vi "带表头写入EXCEL并加入时间量.vi"() -> ()   [LabVIEW 2014]
panel:
  out "保存的路径":path
  out "序号":dbl format="%06.0f"
  in  "起始号":dbl format="%0#6.0p"
  in  "停止":bool
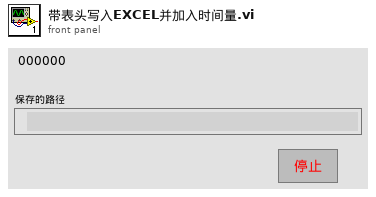
[diagram p1: front panel]
types:
  T1 = enum16{"open", "replace", "create", "open or create", "replace or create", "replace or create with confirmation"}
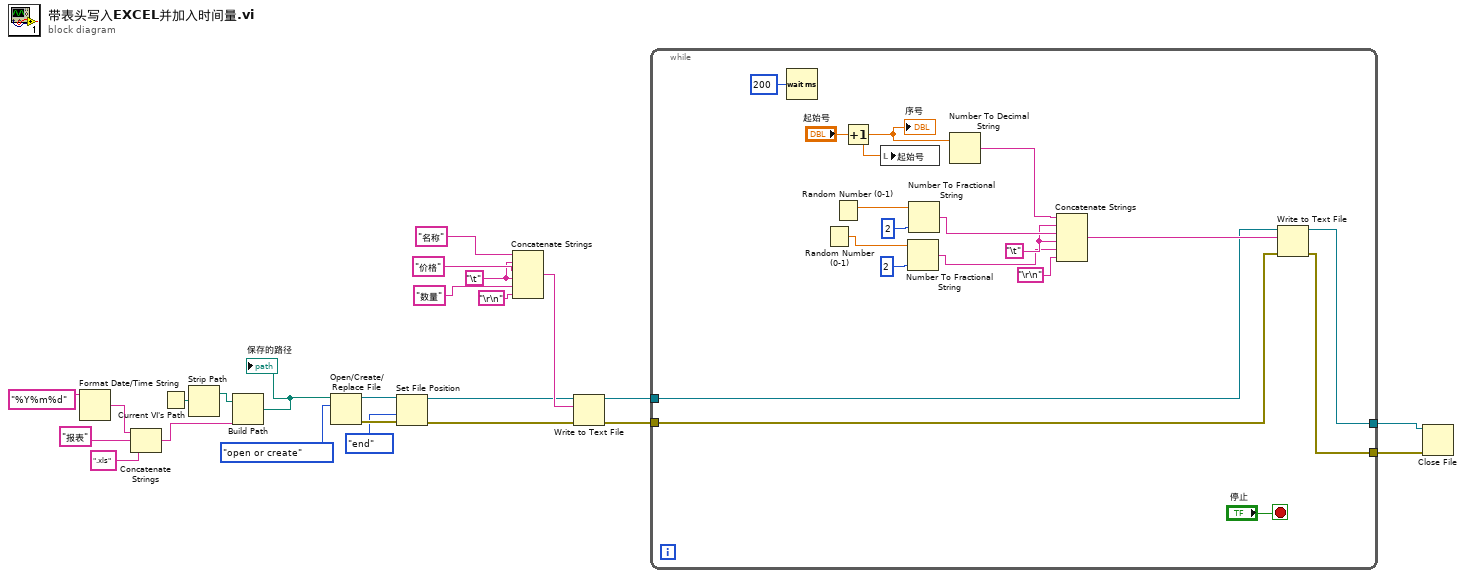
[diagram p0: block diagram]
diagram:
  w5 = "\t"
  n1 = Format Date/Time String(time format string (%c)="%Y%m%d" ("时间格式字符串(%c)")) -> (date/time string=w13:string)  [unwired: 2 in]
  n2 = Concatenate Strings(w13, "报表" ("名称或相对路径"), ".xls" ("字符串")) -> (w19:string)
  n3 = Current VI's Path() -> (path=w18:path)
  n4 = Strip Path(path=w18) -> (stripped path=w17:path)  [unwired: 1 out]
  n5 = Build Path(base path=w17, name or relative path=w19) -> (appended path=w12:path)
  "保存的路径" <- w12
  n6 = Open/Create/Replace File(file path (use dialog)=w12, operation (0:open)=T1."open or create" ("操作(0:open)")) -> (refnum out=w11:refnum<file>, error out=w21:errorcluster)  [unwired: 4 in, 1 out]
  n7 = Set File Position(refnum=w11, from (0:start)=enum16{"start", "end", "current"}."end" ("自（0:起始）"), error in=w21) -> (refnum out=w4:refnum<file>, error out=w3:errorcluster)  [unwired: 1 in]
  n8 = Concatenate Strings("名称" ("字符串"), w5, "价格" ("字符串"), w5, "数量" ("字符串"), "\r\n") -> (w6:string)
  n9 = Write to Text File(file (use dialog)=w4, text=w6, error in=w3) -> (refnum out=w2:refnum<file>, error out=w1:errorcluster)  [unwired: 1 in, 1 out]
  n10 = while {
    tunnel: [w28] -> w24
    tunnel: [w27] -> w23
    tunnel: w2 -> [w26]
    tunnel: w1 -> [w25]
    stop <- "停止" stop-if-true
    w31 = "\t"
    n11 = Wait (ms)(milliseconds to wait=u32 200 ("等待时间（毫秒）")) -> ()  [unwired: 1 out]
    n12 = Random Number (0-1)() -> (number: 0 to 1=w38:dbl)
    n13 = Random Number (0-1)() -> (number: 0 to 1=w36:dbl)
    n14 = Increment(x="起始号") -> (x+1=w34:dbl)
    "序号" <- w34
    n15 = local write "起始号"(w34) -> ()
    n16 = Number To Fractional String(number=w38, precision (6)=i16 2 ("精度(6)")) -> (F-format string=w30:string)  [unwired: 2 in]
    n17 = Number To Fractional String(number=w36, precision (6)=i16 2 ("精度(6)")) -> (F-format string=w32:string)  [unwired: 2 in]
    n18 = Number To Decimal String(number=w34) -> (decimal integer string=w33:string)  [unwired: 1 in]
    n19 = Concatenate Strings(w33, w31, w32, w31, w30, "\r\n") -> (w41:string)
    n20 = Write to Text File(file (use dialog)=w26, text=w41, error in=w25) -> (refnum out=w28:refnum<file>, error out=w27:errorcluster)  [unwired: 1 in, 1 out]
  }
  n21 = Close File(refnum=w24, error in=w23) -> ()  [unwired: 2 out]
